vi "Translation3d_Create_Default.vi"() -> (3 "TRANSLATION3D":T1 {"Z" format="%14.3f"; "Y" format="%14.3f"; "X" format="%14.3f"})   [LabVIEW 2019, in "Trajectory_Library.lvlib"]
doc: "Constructs a Translation2d with the X and Y components equal to the provided values.\n\nRepresents a translation in 2d space. This object can be used to represent a point or a vector.\n\nThis assumes that you are using conventional mathematical axes. When the robot is placed on the origin, facing toward the X direction, moving forward increases the X, whereas moving to the left increases the Y.\n\nParameters:\n - X - The x component of the translation.\n - Y - The y component of the translation.\n\nReturns\n - TRANSLATION - The TRANSLATION data structure"
uses:
  Trajectory_Library.lvlib
  TRANSLATION3D.ctl
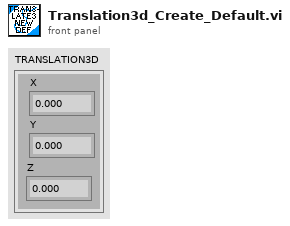
[diagram p1: front panel]
types:
  T1 = typedef "Trajectory_Library.lvlib/TRANSLATION3D.ctl" = cluster{"X":dbl, "Y":dbl, "Z":dbl}
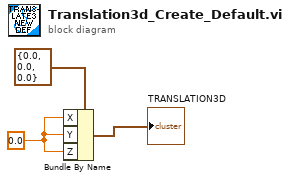
[diagram p0: block diagram]
diagram:
  w2 = 0.0 ("X")
  n1 = Bundle By Name(cluster=T1 {"X"=0.0, "Y"=0.0, "Z"=0.0} ("TRANSLATION"), "X"=w2, "Y"=w2, "Z"=w2) -> (→"TRANSLATION3D":T1)
